vi "Tektronix_scope.vi"(2 "stop":bool, 9 "VISA resource name":refnum<visa-resource-name>) -> ()   [LabVIEW 2020]
doc: "This example illustrates how to use autosetup and continuously acquires waveforms from a single channel using the following steps:\n\n1. Specify a valid VISA session. \n2. Specify a channel. \n3. Specify a time-out value for reading waveform.\n4. Run the VI. The graph displays the waveform you acquire."
uses:
  <instrlib>/Tektronix DPO MSO 2000 4000 Series/Public/Data/Read (Multiple Waveforms).vi
  <vilib>/Waveform/WDTFileIO.llb/Export Waveforms To Spreadsheet File (1D).vi
  <instrlib>/Tektronix DPO MSO 2000 4000 Series/Tektronix DPO MSO 2000 4000 Series.lvlib
panel:
  out "Waveform Graph":waveform(dbl)[](graph)
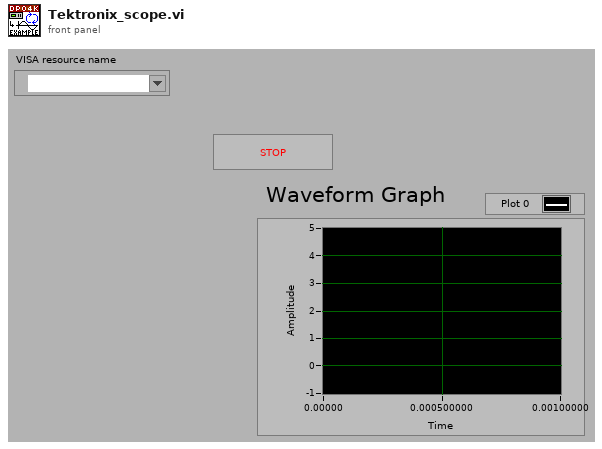
[diagram p1: front panel]
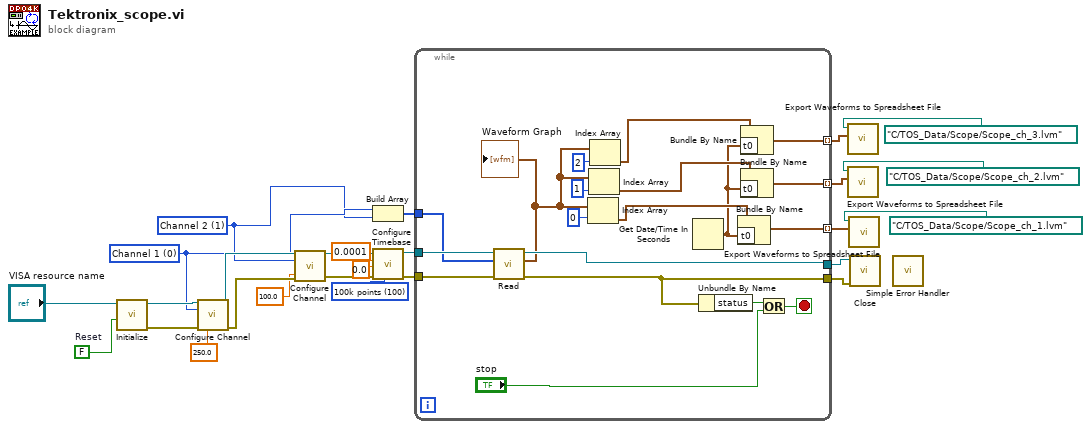
[diagram p0: block diagram]
diagram:
  w13 = u16 1 items=["Channel 1", "Channel 2", "Channel 3", "Channel 4", "Math", "Reference 1", "Reference 2", "Reference 3", "Reference 4", "Bus 1", "Bus 2"] ("Channel (0: Channel 1)")
  w14 = u16 0 items=["Channel 1", "Channel 2", "Channel 3", "Channel 4", "Math", "Reference 1", "Reference 2", "Reference 3", "Reference 4", "Bus 1", "Bus 2"] ("Channel (0: Channel 1)")
  w21 = u32 100 items=["1000 points"=1, "10k points"=10, "100k points"=100, "1M points"=1000, "5M points"=5000, "10M points"=10000] ("Record Length (10: 10k points)")
  w26 = FALSE  # Reset
  n1 = call <instrlib>:"Initialize.vi"("Reset (True)"=w26, "VISA resource name"="VISA resource name") -> ("error out"=w18:errorcluster, "VISA resource name out"=w19:refnum<visa-resource-name>)  [unwired: 8 in]
  n2 = call <instrlib>:"Configure Channel.vi"("VISA resource name"=w19, "Channel (0: Channel 1)"=w14, "error in (no error)"=w18, "Vertical Range (10.0 V)"=250.0) -> ("VISA resource name out"=w17:refnum<visa-resource-name>, "error out"=w16:errorcluster)  [unwired: 10 in]
  n3 = call <instrlib>:"Configure Channel.vi"("VISA resource name"=w17, "Channel (0: Channel 1)"=w13, "error in (no error)"=w16, "Vertical Range (10.0 V)"=100.0) -> ("VISA resource name out"=w7:refnum<visa-resource-name>, "error out"=w8:errorcluster)  [unwired: 10 in]
  n4 = Build Array(w14, w13) -> (w15:u16[])
  n5 = call <instrlib>:"Configure Timebase.vi"("Record Length (10: 10k points)"=w21, "error in (no error)"=w8, "Position (10 %)"=0.0, "Timebase (0.0005 s)"=0.0001, "VISA resource name"=w7) -> ("error out"=w24:errorcluster, "VISA resource name out"=w25:refnum<visa-resource-name>)  [unwired: 5 in]
  n6 = while {
    tunnel: w25 -> [w45]
    tunnel: w24 -> [w44]
    tunnel: [w43] -> w20
    tunnel: w15 -> [w41]
    tunnel: [w38] -> w9
    tunnel: [w35] -> w6 mode=indexing
    tunnel: [w28] -> w5 mode=indexing
    tunnel: [w27] -> w4 mode=indexing
    stop <- w39 stop-if-true
    n7 = call-poly <instrlib>:"Read.vi"("error in (no error)"=w44, "Channels"=w41, "VISA resource name"=w45) -> ("error out"=w38:errorcluster, "Waveform Data"=w32:waveform(dbl)[], "VISA resource name out"=w43:refnum<visa-resource-name>)  [unwired: 6 in]
    "Waveform Graph" <- w32
    n8 = Index Array(array=w32, index=0) -> (element=w36:waveform(dbl))
    n9 = Index Array(array=w32, index=1) -> (element=w30:waveform(dbl))
    n10 = Index Array(array=w32, index=2) -> (element=w31:waveform(dbl))
    n11 = Get Date/Time In Seconds() -> (seconds since 1Jan1904=w29:timestamp)
    n12 = Unbundle By Name(w38) -> ("status"=w42:bool)
    n13 = Bundle By Name(cluster=w36, "t0"=w29) -> (w35:waveform(dbl))
    n14 = Bundle By Name(cluster=w31, "t0"=w29) -> (w27:waveform(dbl))
    n15 = Bundle By Name(cluster=w30, "t0"=w29) -> (w28:waveform(dbl))
    n16 = Or(x=w42, y="stop") -> (x .or. y?=w39:bool)
  }
  n17 = call-poly <vilib>:"Export Waveforms to Spreadsheet File.vi"("waveforms"=w4, "file path (dialog if empty)"=path "C:/TOS_Data/Scope/Scope_ch_3.lvm") -> ()  [unwired: 8 in, 2 out]
  n18 = call-poly <vilib>:"Export Waveforms to Spreadsheet File.vi"("waveforms"=w5, "file path (dialog if empty)"=path "C:/TOS_Data/Scope/Scope_ch_2.lvm") -> ()  [unwired: 8 in, 2 out]
  n19 = call-poly <vilib>:"Export Waveforms to Spreadsheet File.vi"("waveforms"=w6, "file path (dialog if empty)"=path "C:/TOS_Data/Scope/Scope_ch_1.lvm") -> ()  [unwired: 8 in, 2 out]
  n20 = call <instrlib>:"Close.vi"("error in (no error)"=w9, "VISA resource name"=w20) -> ()  [unwired: 9 in, 1 out]
  n21 = call <vilib>:"Simple Error Handler.vi"() -> ()  [unwired: 5 in, 5 out]
